vi "S4GUI_001.vi"() -> ()   [LabVIEW 2018] (continued)
            n2258 = call-dynamic "Write ObsType.vi"("error in (no error)"=w5379, "ObsType"=w5365, "Interface in"=w5373) -> ("error out"=w5378:errorcluster, "Interface out"=w5372:refnum<class "Interface.lvclass">)  [unwired: 7 in]
            n2259 = call-dynamic "Write Object.vi"("error in (no error)"=w5378, "Object"=w5364, "Interface in"=w5372) -> ("error out"=w5377:errorcluster, "Interface out"=w5371:refnum<class "Interface.lvclass">)  [unwired: 7 in]
            n2260 = call-dynamic "Write Comments.vi"("error in (no error)"=w5377, "Comments"=w5366, "Interface in"=w5371) -> ("error out"=w5358:errorcluster, "Interface out"=w5357:refnum<class "Interface.lvclass">)  [unwired: 7 in]
            n2261 = call-dynamic "Write Observer.vi"("error in (no error)"=w5358, "Observer"=w5363, "Interface in"=w5357) -> ("error out"=w5359:errorcluster, "Interface out"=w5360:refnum<class "Interface.lvclass">)  [unwired: 7 in]
            n2262 = call-dynamic "Write Interface.vi"("error in (no error)"=w5359, "Interface.lvclass"=w5360, "Channel in"=w5374) -> ("error out"=w5352:errorcluster, "Channel out"=w5353:refnum<class "Channel.lvclass">)  [unwired: 7 in]
            n2263 = call-dynamic "Read State Machine.vi"("error in (no error)"=w5352, "Device in"=w5353) -> ("error out"=w5356:errorcluster, "State Machine.lvclass"=w5349:refnum<class "State Machine.lvclass">, "Device out"=w5351:refnum<class "Channel.lvclass">)  [unwired: 7 in]
            n2264 = call "Next State.vi"("error in (no error)"=w5356, "New_State"=12, "State Machine in"=w5349) -> ("error out"=w5355:errorcluster, "State Machine out"=w5348:refnum<class "State Machine.lvclass">)  [unwired: 7 in]
            n2265 = call-dynamic "Write State Machine.vi"("error in (no error)"=w5355, "State Machine.lvclass"=w5348, "Device in"=w5351) -> ("error out"=w5347:errorcluster, "Device out"=w5350:refnum<class "Channel.lvclass">)  [unwired: 7 in]
            n2266 = call-dynamic "Write Channel.vi"("error in (no error)"=w5347, "Channel.lvclass"=w5350, "Acquisition in"=w5369) -> ("error out"=w5367:errorcluster, "Acquisition out"=w5368:refnum<class "Acquisition.lvclass">)  [unwired: 7 in]
            n2267 = call-dynamic "Write AcquisitionC.vi"("error in (no error)"=w5367, "Acquisition.lvclass"=w5368, "S4ACS_GUI in"=w5370) -> ("error out"=w5381:errorcluster, "S4ACS_GUI out"=w5382:refnum<class "S4GUI.lvclass">)  [unwired: 7 in]
          }
          frame #3 {
            # "object"
            # "suffix"
            # "obsType"
            n2268 = call-dynamic "Read AcquisitionD.vi"("error in (no error)"=w5426, "S4ACS_GUI in"=w5427) -> ("error out"=w5419:errorcluster, "Acquisition.lvclass"=w5418:refnum<class "Acquisition.lvclass">, "S4ACS_GUI out"=w5413:refnum<class "S4GUI.lvclass">)  [unwired: 7 in]
            n2269 = call-dynamic "Read Channel.vi"("error in (no error)"=w5419, "Acquisition in"=w5418) -> ("error out"=w5386:errorcluster, "Channel.lvclass"=w5388:refnum<class "Channel.lvclass">, "Acquisition out"=w5412:refnum<class "Acquisition.lvclass">)  [unwired: 7 in]
            n2270 = local read "Filter4"() -> (w5389:u8)
            n2271 = call-dynamic "Write Filter.vi"("error in (no error)"=w5386, "Filter"=w5389, "Channel in"=w5388) -> ("error out"=w5385:errorcluster, "Channel out"=w5387:refnum<class "Channel.lvclass">)  [unwired: 7 in]
            n2272 = call-dynamic "Read Interface.vi"("error in (no error)"=w5385, "Channel in"=w5387) -> ("error out"=w5404:errorcluster, "Interface.lvclass"=w5405:refnum<class "Interface.lvclass">, "Channel out"=w5417:refnum<class "Channel.lvclass">)  [unwired: 7 in]
            n2273 = call-dynamic "Write Suffix.vi"("error in (no error)"=w5404, "Suffix"=w5423, "Interface in"=w5405) -> ("error out"=w5422:errorcluster, "Interface out"=w5416:refnum<class "Interface.lvclass">)  [unwired: 7 in]
            n2274 = call-dynamic "Write ObsType.vi"("error in (no error)"=w5422, "ObsType"=w5408, "Interface in"=w5416) -> ("error out"=w5421:errorcluster, "Interface out"=w5415:refnum<class "Interface.lvclass">)  [unwired: 7 in]
            n2275 = call-dynamic "Write Object.vi"("error in (no error)"=w5421, "Object"=w5407, "Interface in"=w5415) -> ("error out"=w5420:errorcluster, "Interface out"=w5414:refnum<class "Interface.lvclass">)  [unwired: 7 in]
            n2276 = call-dynamic "Write Comments.vi"("error in (no error)"=w5420, "Comments"=w5409, "Interface in"=w5414) -> ("error out"=w5403:errorcluster, "Interface out"=w5402:refnum<class "Interface.lvclass">)  [unwired: 7 in]
            n2277 = call-dynamic "Write Observer.vi"("error in (no error)"=w5403, "Observer"=w5406, "Interface in"=w5402) -> ("error out"=w5398:errorcluster, "Interface out"=w5397:refnum<class "Interface.lvclass">)  [unwired: 7 in]
            n2278 = call-dynamic "Write Interface.vi"("error in (no error)"=w5398, "Interface.lvclass"=w5397, "Channel in"=w5417) -> ("error out"=w5393:errorcluster, "Channel out"=w5396:refnum<class "Channel.lvclass">)  [unwired: 7 in]
            n2279 = call-dynamic "Read State Machine.vi"("error in (no error)"=w5393, "Device in"=w5396) -> ("error out"=w5401:errorcluster, "State Machine.lvclass"=w5391:refnum<class "State Machine.lvclass">, "Device out"=w5395:refnum<class "Channel.lvclass">)  [unwired: 7 in]
            n2280 = call "Next State.vi"("error in (no error)"=w5401, "New_State"=12, "State Machine in"=w5391) -> ("error out"=w5400:errorcluster, "State Machine out"=w5390:refnum<class "State Machine.lvclass">)  [unwired: 7 in]
            n2281 = call-dynamic "Write State Machine.vi"("error in (no error)"=w5400, "State Machine.lvclass"=w5390, "Device in"=w5395) -> ("error out"=w5392:errorcluster, "Device out"=w5394:refnum<class "Channel.lvclass">)  [unwired: 7 in]
            n2282 = call-dynamic "Write Channel.vi"("error in (no error)"=w5392, "Channel.lvclass"=w5394, "Acquisition in"=w5412) -> ("error out"=w5410:errorcluster, "Acquisition out"=w5411:refnum<class "Acquisition.lvclass">)  [unwired: 7 in]
            n2283 = call-dynamic "Write AcquisitionD.vi"("error in (no error)"=w5410, "Acquisition.lvclass"=w5411, "S4ACS_GUI in"=w5413) -> ("error out"=w5424:errorcluster, "S4ACS_GUI out"=w5425:refnum<class "S4GUI.lvclass">)  [unwired: 7 in]
          }
        }
      }
      event "object suffix", "dflat suffix", "sflat suffix", "dark suffix", "zero suffix", "focus suffix": Value Change {
        # "Remove todos <\\n> e <space> do sufixo:"
        n2284 = event-data() -> ("NewVal"=w5436:string)  [unwired: 1 in, 5 out]
        n2285 = To Lower Case(string=w5436) -> (all lower case string=w5435:string)
        n2286 = call <vilib>:"Trim Whitespace.vi"("string"=w5435) -> ("trimmed string"=w5434:string)  [unwired: 1 in]
        n2287 = Search and Replace String(replace all?=TRUE ("replace all? (F)"), input string=w5434, search string="\n") -> (result string=w5432:string)  [unwired: 5 in, 3 out]
        n2288 = call <vilib>:"Space Constant.vi"() -> ("String"=w5430:string)
        n2289 = Search and Replace String(replace all?=TRUE ("replace all? (F)"), input string=w5432, search string=w5430) -> (result string=w5433:string)  [unwired: 5 in, 3 out]
        n2290 = stacked-sequence {
          seq-local: [w5472 _ _ _] -> [_ w5530 _ _]
          seq-local: [w5471 _ _ _] -> [_ w5529 _ _]
          seq-local: [_ w5528 _ _] -> [_ _ w5573 _]
          seq-local: [_ w5527 _ _] -> [_ _ w5572 _]
          seq-local: [_ _ w5571 _] -> [_ _ _ w5616]
          seq-local: [_ _ w5570 _] -> [_ _ _ w5615]
          tunnel: w5443 -> [w5484 _ _ _]
          tunnel: w5444 -> [w5483 _ _ _]
          tunnel: [_ _ _ w5614] -> w5438
          tunnel: [_ _ _ w5613] -> w5437
          tunnel: w5433 -> [w5470 w5526 w5569 w5612]
          tunnel: w5441 -> [w5469 w5525 w5555 w5598]
          tunnel: w5439 -> [w5468 w5511 w5554 w5597]
          tunnel: w5442 -> [w5467 w5510 w5553 w5596]
          tunnel: w5440 -> [w5466 w5509 w5552 w5595]
          frame #0 {
            # "observer"
            # "comment"
            # "object"
            # "suffix"
            # "obsType"
            n2291 = call-dynamic "Read AcquisitionA.vi"("error in (no error)"=w5484, "S4ACS_GUI in"=w5483) -> ("error out"=w5482:errorcluster, "Acquisition.lvclass"=w5481:refnum<class "Acquisition.lvclass">, "S4ACS_GUI out"=w5476:refnum<class "S4GUI.lvclass">)  [unwired: 7 in]
            n2292 = call-dynamic "Read Channel.vi"("error in (no error)"=w5482, "Acquisition in"=w5481) -> ("error out"=w5446:errorcluster, "Channel.lvclass"=w5449:refnum<class "Channel.lvclass">, "Acquisition out"=w5475:refnum<class "Acquisition.lvclass">)  [unwired: 7 in]
            n2293 = local read "Filter1"() -> (w5447:u8)
            n2294 = call-dynamic "Write Filter.vi"("error in (no error)"=w5446, "Filter"=w5447, "Channel in"=w5449) -> ("error out"=w5445:errorcluster, "Channel out"=w5448:refnum<class "Channel.lvclass">)  [unwired: 7 in]
            n2295 = call-dynamic "Read Interface.vi"("error in (no error)"=w5445, "Channel in"=w5448) -> ("error out"=w5462:errorcluster, "Interface.lvclass"=w5463:refnum<class "Interface.lvclass">, "Channel out"=w5480:refnum<class "Channel.lvclass">)  [unwired: 7 in]
            n2296 = call-dynamic "Write Suffix.vi"("error in (no error)"=w5462, "Suffix"=w5470, "Interface in"=w5463) -> ("error out"=w5487:errorcluster, "Interface out"=w5479:refnum<class "Interface.lvclass">)  [unwired: 7 in]
            n2297 = call-dynamic "Write ObsType.vi"("error in (no error)"=w5487, "ObsType"=w5468, "Interface in"=w5479) -> ("error out"=w5486:errorcluster, "Interface out"=w5478:refnum<class "Interface.lvclass">)  [unwired: 7 in]
            n2298 = call-dynamic "Write Object.vi"("error in (no error)"=w5486, "Object"=w5467, "Interface in"=w5478) -> ("error out"=w5485:errorcluster, "Interface out"=w5477:refnum<class "Interface.lvclass">)  [unwired: 7 in]
            n2299 = call-dynamic "Write Comments.vi"("error in (no error)"=w5485, "Comments"=w5469, "Interface in"=w5477) -> ("error out"=w5465:errorcluster, "Interface out"=w5464:refnum<class "Interface.lvclass">)  [unwired: 7 in]
            n2300 = call-dynamic "Write Observer.vi"("error in (no error)"=w5465, "Observer"=w5466, "Interface in"=w5464) -> ("error out"=w5460:errorcluster, "Interface out"=w5461:refnum<class "Interface.lvclass">)  [unwired: 7 in]
            n2301 = call-dynamic "Write Interface.vi"("error in (no error)"=w5460, "Interface.lvclass"=w5461, "Channel in"=w5480) -> ("error out"=w5456:errorcluster, "Channel out"=w5459:refnum<class "Channel.lvclass">)  [unwired: 7 in]
            n2302 = call-dynamic "Read State Machine.vi"("error in (no error)"=w5456, "Device in"=w5459) -> ("error out"=w5455:errorcluster, "State Machine.lvclass"=w5453:refnum<class "State Machine.lvclass">, "Device out"=w5458:refnum<class "Channel.lvclass">)  [unwired: 7 in]
            n2303 = call "Next State.vi"("error in (no error)"=w5455, "New_State"=12, "State Machine in"=w5453) -> ("error out"=w5454:errorcluster, "State Machine out"=w5452:refnum<class "State Machine.lvclass">)  [unwired: 7 in]
            n2304 = call-dynamic "Write State Machine.vi"("error in (no error)"=w5454, "State Machine.lvclass"=w5452, "Device in"=w5458) -> ("error out"=w5451:errorcluster, "Device out"=w5457:refnum<class "Channel.lvclass">)  [unwired: 7 in]
            n2305 = call-dynamic "Write Channel.vi"("error in (no error)"=w5451, "Channel.lvclass"=w5457, "Acquisition in"=w5475) -> ("error out"=w5473:errorcluster, "Acquisition out"=w5474:refnum<class "Acquisition.lvclass">)  [unwired: 7 in]
            n2306 = call-dynamic "Write AcquisitionA.vi"("error in (no error)"=w5473, "Acquisition.lvclass"=w5474, "S4ACS_GUI in"=w5476) -> ("error out"=w5471:errorcluster, "S4ACS_GUI out"=w5472:refnum<class "S4GUI.lvclass">)  [unwired: 7 in]
          }
          frame #1 {
            # "object"
            # "suffix"
            # "obsType"
            n2307 = call "Read AcquisitionB.vi"("error in (no error)"=w5529, "S4ACS_GUI in"=w5530) -> ("error out"=w5515:errorcluster, "Acquisition.lvclass"=w5516:refnum<class "Acquisition.lvclass">, "S4ACS_GUI out"=w5521:refnum<class "S4GUI.lvclass">)  [unwired: 7 in]
            n2308 = call-dynamic "Read Channel.vi"("error in (no error)"=w5515, "Acquisition in"=w5516) -> ("error out"=w5489:errorcluster, "Channel.lvclass"=w5491:refnum<class "Channel.lvclass">, "Acquisition out"=w5522:refnum<class "Acquisition.lvclass">)  [unwired: 7 in]
            n2309 = local read "Filter2"() -> (w5492:u8)
            n2310 = call-dynamic "Write Filter.vi"("error in (no error)"=w5489, "Filter"=w5492, "Channel in"=w5491) -> ("error out"=w5488:errorcluster, "Channel out"=w5490:refnum<class "Channel.lvclass">)  [unwired: 7 in]
            n2311 = call-dynamic "Read Interface.vi"("error in (no error)"=w5488, "Channel in"=w5490) -> ("error out"=w5503:errorcluster, "Interface.lvclass"=w5504:refnum<class "Interface.lvclass">, "Channel out"=w5517:refnum<class "Channel.lvclass">)  [unwired: 7 in]
            n2312 = call-dynamic "Write Suffix.vi"("error in (no error)"=w5503, "Suffix"=w5526, "Interface in"=w5504) -> ("error out"=w5512:errorcluster, "Interface out"=w5518:refnum<class "Interface.lvclass">)  [unwired: 7 in]
            n2313 = call-dynamic "Write ObsType.vi"("error in (no error)"=w5512, "ObsType"=w5511, "Interface in"=w5518) -> ("error out"=w5513:errorcluster, "Interface out"=w5519:refnum<class "Interface.lvclass">)  [unwired: 7 in]
            n2314 = call-dynamic "Write Object.vi"("error in (no error)"=w5513, "Object"=w5510, "Interface in"=w5519) -> ("error out"=w5514:errorcluster, "Interface out"=w5520:refnum<class "Interface.lvclass">)  [unwired: 7 in]
            n2315 = call-dynamic "Write Comments.vi"("error in (no error)"=w5514, "Comments"=w5525, "Interface in"=w5520) -> ("error out"=w5506:errorcluster, "Interface out"=w5505:refnum<class "Interface.lvclass">)  [unwired: 7 in]
            n2316 = call-dynamic "Write Observer.vi"("error in (no error)"=w5506, "Observer"=w5509, "Interface in"=w5505) -> ("error out"=w5507:errorcluster, "Interface out"=w5508:refnum<class "Interface.lvclass">)  [unwired: 7 in]
            n2317 = call-dynamic "Write Interface.vi"("error in (no error)"=w5507, "Interface.lvclass"=w5508, "Channel in"=w5517) -> ("error out"=w5496:errorcluster, "Channel out"=w5497:refnum<class "Channel.lvclass">)  [unwired: 7 in]
            n2318 = call-dynamic "Read State Machine.vi"("error in (no error)"=w5496, "Device in"=w5497) -> ("error out"=w5502:errorcluster, "State Machine.lvclass"=w5500:refnum<class "State Machine.lvclass">, "Device out"=w5495:refnum<class "Channel.lvclass">)  [unwired: 7 in]
            n2319 = call "Next State.vi"("error in (no error)"=w5502, "New_State"=12, "State Machine in"=w5500) -> ("error out"=w5501:errorcluster, "State Machine out"=w5499:refnum<class "State Machine.lvclass">)  [unwired: 7 in]
            n2320 = call-dynamic "Write State Machine.vi"("error in (no error)"=w5501, "State Machine.lvclass"=w5499, "Device in"=w5495) -> ("error out"=w5493:errorcluster, "Device out"=w5494:refnum<class "Channel.lvclass">)  [unwired: 7 in]
            n2321 = call-dynamic "Write Channel.vi"("error in (no error)"=w5493, "Channel.lvclass"=w5494, "Acquisition in"=w5522) -> ("error out"=w5524:errorcluster, "Acquisition out"=w5523:refnum<class "Acquisition.lvclass">)  [unwired: 7 in]
            n2322 = call "Write AcquisitionB.vi"("error in (no error)"=w5524, "Acquisition.lvclass"=w5523, "S4ACS_GUI in"=w5521) -> ("error out"=w5527:errorcluster, "S4ACS_GUI out"=w5528:refnum<class "S4GUI.lvclass">)  [unwired: 7 in]
          }
          frame #2 {
            # "object"
            # "suffix"
            # "obsType"
            n2323 = call-dynamic "Read AcquisitionC.vi"("error in (no error)"=w5572, "S4ACS_GUI in"=w5573) -> ("error out"=w5565:errorcluster, "Acquisition.lvclass"=w5564:refnum<class "Acquisition.lvclass">, "S4ACS_GUI out"=w5559:refnum<class "S4GUI.lvclass">)  [unwired: 7 in]
            n2324 = call-dynamic "Read Channel.vi"("error in (no error)"=w5565, "Acquisition in"=w5564) -> ("error out"=w5532:errorcluster, "Channel.lvclass"=w5534:refnum<class "Channel.lvclass">, "Acquisition out"=w5558:refnum<class "Acquisition.lvclass">)  [unwired: 7 in]
            n2325 = local read "Filter3"() -> (w5535:u8)
            n2326 = call-dynamic "Write Filter.vi"("error in (no error)"=w5532, "Filter"=w5535, "Channel in"=w5534) -> ("error out"=w5531:errorcluster, "Channel out"=w5533:refnum<class "Channel.lvclass">)  [unwired: 7 in]
            n2327 = call-dynamic "Read Interface.vi"("error in (no error)"=w5531, "Channel in"=w5533) -> ("error out"=w5550:errorcluster, "Interface.lvclass"=w5551:refnum<class "Interface.lvclass">, "Channel out"=w5563:refnum<class "Channel.lvclass">)  [unwired: 7 in]
            n2328 = call-dynamic "Write Suffix.vi"("error in (no error)"=w5550, "Suffix"=w5569, "Interface in"=w5551) -> ("error out"=w5568:errorcluster, "Interface out"=w5562:refnum<class "Interface.lvclass">)  [unwired: 7 in]
            n2329 = call-dynamic "Write ObsType.vi"("error in (no error)"=w5568, "ObsType"=w5554, "Interface in"=w5562) -> ("error out"=w5567:errorcluster, "Interface out"=w5561:refnum<class "Interface.lvclass">)  [unwired: 7 in]
            n2330 = call-dynamic "Write Object.vi"("error in (no error)"=w5567, "Object"=w5553, "Interface in"=w5561) -> ("error out"=w5566:errorcluster, "Interface out"=w5560:refnum<class "Interface.lvclass">)  [unwired: 7 in]
            n2331 = call-dynamic "Write Comments.vi"("error in (no error)"=w5566, "Comments"=w5555, "Interface in"=w5560) -> ("error out"=w5547:errorcluster, "Interface out"=w5546:refnum<class "Interface.lvclass">)  [unwired: 7 in]
            n2332 = call-dynamic "Write Observer.vi"("error in (no error)"=w5547, "Observer"=w5552, "Interface in"=w5546) -> ("error out"=w5548:errorcluster, "Interface out"=w5549:refnum<class "Interface.lvclass">)  [unwired: 7 in]
            n2333 = call-dynamic "Write Interface.vi"("error in (no error)"=w5548, "Interface.lvclass"=w5549, "Channel in"=w5563) -> ("error out"=w5541:errorcluster, "Channel out"=w5542:refnum<class "Channel.lvclass">)  [unwired: 7 in]
            n2334 = call-dynamic "Read State Machine.vi"("error in (no error)"=w5541, "Device in"=w5542) -> ("error out"=w5545:errorcluster, "State Machine.lvclass"=w5538:refnum<class "State Machine.lvclass">, "Device out"=w5540:refnum<class "Channel.lvclass">)  [unwired: 7 in]
            n2335 = call "Next State.vi"("error in (no error)"=w5545, "New_State"=12, "State Machine in"=w5538) -> ("error out"=w5544:errorcluster, "State Machine out"=w5537:refnum<class "State Machine.lvclass">)  [unwired: 7 in]
            n2336 = call-dynamic "Write State Machine.vi"("error in (no error)"=w5544, "State Machine.lvclass"=w5537, "Device in"=w5540) -> ("error out"=w5536:errorcluster, "Device out"=w5539:refnum<class "Channel.lvclass">)  [unwired: 7 in]
            n2337 = call-dynamic "Write Channel.vi"("error in (no error)"=w5536, "Channel.lvclass"=w5539, "Acquisition in"=w5558) -> ("error out"=w5556:errorcluster, "Acquisition out"=w5557:refnum<class "Acquisition.lvclass">)  [unwired: 7 in]
            n2338 = call-dynamic "Write AcquisitionC.vi"("error in (no error)"=w5556, "Acquisition.lvclass"=w5557, "S4ACS_GUI in"=w5559) -> ("error out"=w5570:errorcluster, "S4ACS_GUI out"=w5571:refnum<class "S4GUI.lvclass">)  [unwired: 7 in]
          }
          frame #3 {
            # "object"
            # "suffix"
            # "obsType"
            n2339 = call-dynamic "Read AcquisitionD.vi"("error in (no error)"=w5615, "S4ACS_GUI in"=w5616) -> ("error out"=w5608:errorcluster, "Acquisition.lvclass"=w5607:refnum<class "Acquisition.lvclass">, "S4ACS_GUI out"=w5602:refnum<class "S4GUI.lvclass">)  [unwired: 7 in]
            n2340 = call-dynamic "Read Channel.vi"("error in (no error)"=w5608, "Acquisition in"=w5607) -> ("error out"=w5575:errorcluster, "Channel.lvclass"=w5577:refnum<class "Channel.lvclass">, "Acquisition out"=w5601:refnum<class "Acquisition.lvclass">)  [unwired: 7 in]
            n2341 = local read "Filter4"() -> (w5578:u8)
            n2342 = call-dynamic "Write Filter.vi"("error in (no error)"=w5575, "Filter"=w5578, "Channel in"=w5577) -> ("error out"=w5574:errorcluster, "Channel out"=w5576:refnum<class "Channel.lvclass">)  [unwired: 7 in]
            n2343 = call-dynamic "Read Interface.vi"("error in (no error)"=w5574, "Channel in"=w5576) -> ("error out"=w5593:errorcluster, "Interface.lvclass"=w5594:refnum<class "Interface.lvclass">, "Channel out"=w5606:refnum<class "Channel.lvclass">)  [unwired: 7 in]
            n2344 = call-dynamic "Write Suffix.vi"("error in (no error)"=w5593, "Suffix"=w5612, "Interface in"=w5594) -> ("error out"=w5611:errorcluster, "Interface out"=w5605:refnum<class "Interface.lvclass">)  [unwired: 7 in]
            n2345 = call-dynamic "Write ObsType.vi"("error in (no error)"=w5611, "ObsType"=w5597, "Interface in"=w5605) -> ("error out"=w5610:errorcluster, "Interface out"=w5604:refnum<class "Interface.lvclass">)  [unwired: 7 in]
            n2346 = call-dynamic "Write Object.vi"("error in (no error)"=w5610, "Object"=w5596, "Interface in"=w5604) -> ("error out"=w5609:errorcluster, "Interface out"=w5603:refnum<class "Interface.lvclass">)  [unwired: 7 in]
            n2347 = call-dynamic "Write Comments.vi"("error in (no error)"=w5609, "Comments"=w5598, "Interface in"=w5603) -> ("error out"=w5592:errorcluster, "Interface out"=w5591:refnum<class "Interface.lvclass">)  [unwired: 7 in]
            n2348 = call-dynamic "Write Observer.vi"("error in (no error)"=w5592, "Observer"=w5595, "Interface in"=w5591) -> ("error out"=w5587:errorcluster, "Interface out"=w5586:refnum<class "Interface.lvclass">)  [unwired: 7 in]
            n2349 = call-dynamic "Write Interface.vi"("error in (no error)"=w5587, "Interface.lvclass"=w5586, "Channel in"=w5606) -> ("error out"=w5582:errorcluster, "Channel out"=w5585:refnum<class "Channel.lvclass">)  [unwired: 7 in]
            n2350 = call-dynamic "Read State Machine.vi"("error in (no error)"=w5582, "Device in"=w5585) -> ("error out"=w5590:errorcluster, "State Machine.lvclass"=w5580:refnum<class "State Machine.lvclass">, "Device out"=w5584:refnum<class "Channel.lvclass">)  [unwired: 7 in]
            n2351 = call "Next State.vi"("error in (no error)"=w5590, "New_State"=12, "State Machine in"=w5580) -> ("error out"=w5589:errorcluster, "State Machine out"=w5579:refnum<class "State Machine.lvclass">)  [unwired: 7 in]
            n2352 = call-dynamic "Write State Machine.vi"("error in (no error)"=w5589, "State Machine.lvclass"=w5579, "Device in"=w5584) -> ("error out"=w5581:errorcluster, "Device out"=w5583:refnum<class "Channel.lvclass">)  [unwired: 7 in]
            n2353 = call-dynamic "Write Channel.vi"("error in (no error)"=w5581, "Channel.lvclass"=w5583, "Acquisition in"=w5601) -> ("error out"=w5599:errorcluster, "Acquisition out"=w5600:refnum<class "Acquisition.lvclass">)  [unwired: 7 in]
            n2354 = call-dynamic "Write AcquisitionD.vi"("error in (no error)"=w5599, "Acquisition.lvclass"=w5600, "S4ACS_GUI in"=w5602) -> ("error out"=w5613:errorcluster, "S4ACS_GUI out"=w5614:refnum<class "S4GUI.lvclass">)  [unwired: 7 in]
          }
        }
      }
      event "Observer": Value Change {
        n2355 = event-data() -> ("NewVal"=w5617:string)  [unwired: 1 in, 5 out]
        n2356 = disable-structure shown="Enabled" {
          disable-tunnel: w5620 -> [w5635 w5636]
          disable-tunnel: w5617 -> [w5634 _]
          disable-tunnel: [w5633 w5636] -> w5619
          frame Disabled {
            n2357 = String Length(string=w5634) -> (length=w5632:i32)
            n2358 = Equal To 0?(x=w5632) -> (x = 0?=w5631:bool)
            n2359 = Select(t=u32 16777216, s=w5631, f=u32 16777225) -> (s? t:f=w5629:u32)
            n2360 = property on="Observer" class="Str"(error in=w5635, "Text.BGColor"=w5629) -> (error out=w5633:errorcluster)  [unwired: 1 in, 1 out]
          }
          frame Enabled {
            # "Não se usa mais o texto de fundo\ndo controle \"Observer\""
          }
        }
        n2361 = case shown="False" FALSE {
          tunnel: w5627 -> [w5645 w5819]
          tunnel: w5626 -> [w5644 _]
          tunnel: w5625 -> [w5643 _]
          tunnel: w5624 -> [w5642 _]
          tunnel: w5617 -> [w5641 _]
          tunnel: w5623 -> [w5640 _]
          tunnel: [w5639 w5819] -> w5622
          tunnel: [w5638 w5818] -> w5621
          tunnel: w5619 -> [w5637 w5818]
          frame False {
            n2362 = stacked-sequence {
              seq-local: [w5673 _ _ _] -> [_ w5731 _ _]
              seq-local: [w5672 _ _ _] -> [_ w5730 _ _]
              seq-local: [_ w5729 _ _] -> [_ _ w5774 _]
              seq-local: [_ w5728 _ _] -> [_ _ w5773 _]
              seq-local: [_ _ w5772 _] -> [_ _ _ w5817]
              seq-local: [_ _ w5771 _] -> [_ _ _ w5816]
              tunnel: w5637 -> [w5685 _ _ _]
              tunnel: w5645 -> [w5684 _ _ _]
              tunnel: [_ _ _ w5815] -> w5639
              tunnel: [_ _ _ w5814] -> w5638
              tunnel: w5643 -> [w5671 w5727 w5770 w5813]
              tunnel: w5642 -> [w5670 w5726 w5756 w5799]
              tunnel: w5640 -> [w5669 w5712 w5755 w5798]
              tunnel: w5644 -> [w5668 w5711 w5754 w5797]
              tunnel: w5641 -> [w5667 w5710 w5753 w5796]
              frame #0 {
                # "observer"
                # "comment"
                # "object"
                # "suffix"
                # "obsType"
                n2363 = call-dynamic "Read AcquisitionA.vi"("error in (no error)"=w5685, "S4ACS_GUI in"=w5684) -> ("error out"=w5683:errorcluster, "Acquisition.lvclass"=w5682:refnum<class "Acquisition.lvclass">, "S4ACS_GUI out"=w5677:refnum<class "S4GUI.lvclass">)  [unwired: 7 in]
                n2364 = call-dynamic "Read Channel.vi"("error in (no error)"=w5683, "Acquisition in"=w5682) -> ("error out"=w5647:errorcluster, "Channel.lvclass"=w5650:refnum<class "Channel.lvclass">, "Acquisition out"=w5676:refnum<class "Acquisition.lvclass">)  [unwired: 7 in]
                n2365 = local read "Filter1"() -> (w5648:u8)
                n2366 = call-dynamic "Write Filter.vi"("error in (no error)"=w5647, "Filter"=w5648, "Channel in"=w5650) -> ("error out"=w5646:errorcluster, "Channel out"=w5649:refnum<class "Channel.lvclass">)  [unwired: 7 in]
                n2367 = call-dynamic "Read Interface.vi"("error in (no error)"=w5646, "Channel in"=w5649) -> ("error out"=w5663:errorcluster, "Interface.lvclass"=w5664:refnum<class "Interface.lvclass">, "Channel out"=w5681:refnum<class "Channel.lvclass">)  [unwired: 7 in]
                n2368 = call-dynamic "Write Suffix.vi"("error in (no error)"=w5663, "Suffix"=w5671, "Interface in"=w5664) -> ("error out"=w5688:errorcluster, "Interface out"=w5680:refnum<class "Interface.lvclass">)  [unwired: 7 in]
                n2369 = call-dynamic "Write ObsType.vi"("error in (no error)"=w5688, "ObsType"=w5669, "Interface in"=w5680) -> ("error out"=w5687:errorcluster, "Interface out"=w5679:refnum<class "Interface.lvclass">)  [unwired: 7 in]
                n2370 = call-dynamic "Write Object.vi"("error in (no error)"=w5687, "Object"=w5668, "Interface in"=w5679) -> ("error out"=w5686:errorcluster, "Interface out"=w5678:refnum<class "Interface.lvclass">)  [unwired: 7 in]
                n2371 = call-dynamic "Write Comments.vi"("error in (no error)"=w5686, "Comments"=w5670, "Interface in"=w5678) -> ("error out"=w5666:errorcluster, "Interface out"=w5665:refnum<class "Interface.lvclass">)  [unwired: 7 in]
                n2372 = call-dynamic "Write Observer.vi"("error in (no error)"=w5666, "Observer"=w5667, "Interface in"=w5665) -> ("error out"=w5661:errorcluster, "Interface out"=w5662:refnum<class "Interface.lvclass">)  [unwired: 7 in]
                n2373 = call-dynamic "Write Interface.vi"("error in (no error)"=w5661, "Interface.lvclass"=w5662, "Channel in"=w5681) -> ("error out"=w5657:errorcluster, "Channel out"=w5660:refnum<class "Channel.lvclass">)  [unwired: 7 in]
                n2374 = call-dynamic "Read State Machine.vi"("error in (no error)"=w5657, "Device in"=w5660) -> ("error out"=w5656:errorcluster, "State Machine.lvclass"=w5654:refnum<class "State Machine.lvclass">, "Device out"=w5659:refnum<class "Channel.lvclass">)  [unwired: 7 in]
                n2375 = call "Next State.vi"("error in (no error)"=w5656, "New_State"=12, "State Machine in"=w5654) -> ("error out"=w5655:errorcluster, "State Machine out"=w5653:refnum<class "State Machine.lvclass">)  [unwired: 7 in]
                n2376 = call-dynamic "Write State Machine.vi"("error in (no error)"=w5655, "State Machine.lvclass"=w5653, "Device in"=w5659) -> ("error out"=w5652:errorcluster, "Device out"=w5658:refnum<class "Channel.lvclass">)  [unwired: 7 in]
                n2377 = call-dynamic "Write Channel.vi"("error in (no error)"=w5652, "Channel.lvclass"=w5658, "Acquisition in"=w5676) -> ("error out"=w5674:errorcluster, "Acquisition out"=w5675:refnum<class "Acquisition.lvclass">)  [unwired: 7 in]
                n2378 = call-dynamic "Write AcquisitionA.vi"("error in (no error)"=w5674, "Acquisition.lvclass"=w5675, "S4ACS_GUI in"=w5677) -> ("error out"=w5672:errorcluster, "S4ACS_GUI out"=w5673:refnum<class "S4GUI.lvclass">)  [unwired: 7 in]
              }
              frame #1 {
                # "object"
                # "suffix"
                # "obsType"
                n2379 = call "Read AcquisitionB.vi"("error in (no error)"=w5730, "S4ACS_GUI in"=w5731) -> ("error out"=w5716:errorcluster, "Acquisition.lvclass"=w5717:refnum<class "Acquisition.lvclass">, "S4ACS_GUI out"=w5722:refnum<class "S4GUI.lvclass">)  [unwired: 7 in]
                n2380 = call-dynamic "Read Channel.vi"("error in (no error)"=w5716, "Acquisition in"=w5717) -> ("error out"=w5690:errorcluster, "Channel.lvclass"=w5692:refnum<class "Channel.lvclass">, "Acquisition out"=w5723:refnum<class "Acquisition.lvclass">)  [unwired: 7 in]
                n2381 = local read "Filter2"() -> (w5693:u8)
                n2382 = call-dynamic "Write Filter.vi"("error in (no error)"=w5690, "Filter"=w5693, "Channel in"=w5692) -> ("error out"=w5689:errorcluster, "Channel out"=w5691:refnum<class "Channel.lvclass">)  [unwired: 7 in]
                n2383 = call-dynamic "Read Interface.vi"("error in (no error)"=w5689, "Channel in"=w5691) -> ("error out"=w5704:errorcluster, "Interface.lvclass"=w5705:refnum<class "Interface.lvclass">, "Channel out"=w5718:refnum<class "Channel.lvclass">)  [unwired: 7 in]
                n2384 = call-dynamic "Write Suffix.vi"("error in (no error)"=w5704, "Suffix"=w5727, "Interface in"=w5705) -> ("error out"=w5713:errorcluster, "Interface out"=w5719:refnum<class "Interface.lvclass">)  [unwired: 7 in]
                n2385 = call-dynamic "Write ObsType.vi"("error in (no error)"=w5713, "ObsType"=w5712, "Interface in"=w5719) -> ("error out"=w5714:errorcluster, "Interface out"=w5720:refnum<class "Interface.lvclass">)  [unwired: 7 in]
                n2386 = call-dynamic "Write Object.vi"("error in (no error)"=w5714, "Object"=w5711, "Interface in"=w5720) -> ("error out"=w5715:errorcluster, "Interface out"=w5721:refnum<class "Interface.lvclass">)  [unwired: 7 in]
                n2387 = call-dynamic "Write Comments.vi"("error in (no error)"=w5715, "Comments"=w5726, "Interface in"=w5721) -> ("error out"=w5707:errorcluster, "Interface out"=w5706:refnum<class "Interface.lvclass">)  [unwired: 7 in]
                n2388 = call-dynamic "Write Observer.vi"("error in (no error)"=w5707, "Observer"=w5710, "Interface in"=w5706) -> ("error out"=w5708:errorcluster, "Interface out"=w5709:refnum<class "Interface.lvclass">)  [unwired: 7 in]
                n2389 = call-dynamic "Write Interface.vi"("error in (no error)"=w5708, "Interface.lvclass"=w5709, "Channel in"=w5718) -> ("error out"=w5697:errorcluster, "Channel out"=w5698:refnum<class "Channel.lvclass">)  [unwired: 7 in]
                n2390 = call-dynamic "Read State Machine.vi"("error in (no error)"=w5697, "Device in"=w5698) -> ("error out"=w5703:errorcluster, "State Machine.lvclass"=w5701:refnum<class "State Machine.lvclass">, "Device out"=w5696:refnum<class "Channel.lvclass">)  [unwired: 7 in]
                n2391 = call "Next State.vi"("error in (no error)"=w5703, "New_State"=12, "State Machine in"=w5701) -> ("error out"=w5702:errorcluster, "State Machine out"=w5700:refnum<class "State Machine.lvclass">)  [unwired: 7 in]
                n2392 = call-dynamic "Write State Machine.vi"("error in (no error)"=w5702, "State Machine.lvclass"=w5700, "Device in"=w5696) -> ("error out"=w5694:errorcluster, "Device out"=w5695:refnum<class "Channel.lvclass">)  [unwired: 7 in]
                n2393 = call-dynamic "Write Channel.vi"("error in (no error)"=w5694, "Channel.lvclass"=w5695, "Acquisition in"=w5723) -> ("error out"=w5725:errorcluster, "Acquisition out"=w5724:refnum<class "Acquisition.lvclass">)  [unwired: 7 in]
                n2394 = call "Write AcquisitionB.vi"("error in (no error)"=w5725, "Acquisition.lvclass"=w5724, "S4ACS_GUI in"=w5722) -> ("error out"=w5728:errorcluster, "S4ACS_GUI out"=w5729:refnum<class "S4GUI.lvclass">)  [unwired: 7 in]
              }
              frame #2 {
                # "object"
                # "suffix"
                # "obsType"
                n2395 = call-dynamic "Read AcquisitionC.vi"("error in (no error)"=w5773, "S4ACS_GUI in"=w5774) -> ("error out"=w5766:errorcluster, "Acquisition.lvclass"=w5765:refnum<class "Acquisition.lvclass">, "S4ACS_GUI out"=w5760:refnum<class "S4GUI.lvclass">)  [unwired: 7 in]
                n2396 = call-dynamic "Read Channel.vi"("error in (no error)"=w5766, "Acquisition in"=w5765) -> ("error out"=w5733:errorcluster, "Channel.lvclass"=w5735:refnum<class "Channel.lvclass">, "Acquisition out"=w5759:refnum<class "Acquisition.lvclass">)  [unwired: 7 in]
                n2397 = local read "Filter3"() -> (w5736:u8)
                n2398 = call-dynamic "Write Filter.vi"("error in (no error)"=w5733, "Filter"=w5736, "Channel in"=w5735) -> ("error out"=w5732:errorcluster, "Channel out"=w5734:refnum<class "Channel.lvclass">)  [unwired: 7 in]
                n2399 = call-dynamic "Read Interface.vi"("error in (no error)"=w5732, "Channel in"=w5734) -> ("error out"=w5751:errorcluster, "Interface.lvclass"=w5752:refnum<class "Interface.lvclass">, "Channel out"=w5764:refnum<class "Channel.lvclass">)  [unwired: 7 in]
                n2400 = call-dynamic "Write Suffix.vi"("error in (no error)"=w5751, "Suffix"=w5770, "Interface in"=w5752) -> ("error out"=w5769:errorcluster, "Interface out"=w5763:refnum<class "Interface.lvclass">)  [unwired: 7 in]
                n2401 = call-dynamic "Write ObsType.vi"("error in (no error)"=w5769, "ObsType"=w5755, "Interface in"=w5763) -> ("error out"=w5768:errorcluster, "Interface out"=w5762:refnum<class "Interface.lvclass">)  [unwired: 7 in]
                n2402 = call-dynamic "Write Object.vi"("error in (no error)"=w5768, "Object"=w5754, "Interface in"=w5762) -> ("error out"=w5767:errorcluster, "Interface out"=w5761:refnum<class "Interface.lvclass">)  [unwired: 7 in]
                n2403 = call-dynamic "Write Comments.vi"("error in (no error)"=w5767, "Comments"=w5756, "Interface in"=w5761) -> ("error out"=w5748:errorcluster, "Interface out"=w5747:refnum<class "Interface.lvclass">)  [unwired: 7 in]
                n2404 = call-dynamic "Write Observer.vi"("error in (no error)"=w5748, "Observer"=w5753, "Interface in"=w5747) -> ("error out"=w5749:errorcluster, "Interface out"=w5750:refnum<class "Interface.lvclass">)  [unwired: 7 in]
                n2405 = call-dynamic "Write Interface.vi"("error in (no error)"=w5749, "Interface.lvclass"=w5750, "Channel in"=w5764) -> ("error out"=w5742:errorcluster, "Channel out"=w5743:refnum<class "Channel.lvclass">)  [unwired: 7 in]
                n2406 = call-dynamic "Read State Machine.vi"("error in (no error)"=w5742, "Device in"=w5743) -> ("error out"=w5746:errorcluster, "State Machine.lvclass"=w5739:refnum<class "State Machine.lvclass">, "Device out"=w5741:refnum<class "Channel.lvclass">)  [unwired: 7 in]
                n2407 = call "Next State.vi"("error in (no error)"=w5746, "New_State"=12, "State Machine in"=w5739) -> ("error out"=w5745:errorcluster, "State Machine out"=w5738:refnum<class "State Machine.lvclass">)  [unwired: 7 in]
                n2408 = call-dynamic "Write State Machine.vi"("error in (no error)"=w5745, "State Machine.lvclass"=w5738, "Device in"=w5741) -> ("error out"=w5737:errorcluster, "Device out"=w5740:refnum<class "Channel.lvclass">)  [unwired: 7 in]
                n2409 = call-dynamic "Write Channel.vi"("error in (no error)"=w5737, "Channel.lvclass"=w5740, "Acquisition in"=w5759) -> ("error out"=w5757:errorcluster, "Acquisition out"=w5758:refnum<class "Acquisition.lvclass">)  [unwired: 7 in]
                n2410 = call-dynamic "Write AcquisitionC.vi"("error in (no error)"=w5757, "Acquisition.lvclass"=w5758, "S4ACS_GUI in"=w5760) -> ("error out"=w5771:errorcluster, "S4ACS_GUI out"=w5772:refnum<class "S4GUI.lvclass">)  [unwired: 7 in]
              }
              frame #3 {
                # "object"
                # "suffix"
                # "obsType"
                n2411 = call-dynamic "Read AcquisitionD.vi"("error in (no error)"=w5816, "S4ACS_GUI in"=w5817) -> ("error out"=w5809:errorcluster, "Acquisition.lvclass"=w5808:refnum<class "Acquisition.lvclass">, "S4ACS_GUI out"=w5803:refnum<class "S4GUI.lvclass">)  [unwired: 7 in]
                n2412 = call-dynamic "Read Channel.vi"("error in (no error)"=w5809, "Acquisition in"=w5808) -> ("error out"=w5776:errorcluster, "Channel.lvclass"=w5778:refnum<class "Channel.lvclass">, "Acquisition out"=w5802:refnum<class "Acquisition.lvclass">)  [unwired: 7 in]
                n2413 = local read "Filter4"() -> (w5779:u8)
                n2414 = call-dynamic "Write Filter.vi"("error in (no error)"=w5776, "Filter"=w5779, "Channel in"=w5778) -> ("error out"=w5775:errorcluster, "Channel out"=w5777:refnum<class "Channel.lvclass">)  [unwired: 7 in]
                n2415 = call-dynamic "Read Interface.vi"("error in (no error)"=w5775, "Channel in"=w5777) -> ("error out"=w5794:errorcluster, "Interface.lvclass"=w5795:refnum<class "Interface.lvclass">, "Channel out"=w5807:refnum<class "Channel.lvclass">)  [unwired: 7 in]
                n2416 = call-dynamic "Write Suffix.vi"("error in (no error)"=w5794, "Suffix"=w5813, "Interface in"=w5795) -> ("error out"=w5812:errorcluster, "Interface out"=w5806:refnum<class "Interface.lvclass">)  [unwired: 7 in]
                n2417 = call-dynamic "Write ObsType.vi"("error in (no error)"=w5812, "ObsType"=w5798, "Interface in"=w5806) -> ("error out"=w5811:errorcluster, "Interface out"=w5805:refnum<class "Interface.lvclass">)  [unwired: 7 in]
                n2418 = call-dynamic "Write Object.vi"("error in (no error)"=w5811, "Object"=w5797, "Interface in"=w5805) -> ("error out"=w5810:errorcluster, "Interface out"=w5804:refnum<class "Interface.lvclass">)  [unwired: 7 in]
                n2419 = call-dynamic "Write Comments.vi"("error in (no error)"=w5810, "Comments"=w5799, "Interface in"=w5804) -> ("error out"=w5793:errorcluster, "Interface out"=w5792:refnum<class "Interface.lvclass">)  [unwired: 7 in]
                n2420 = call-dynamic "Write Observer.vi"("error in (no error)"=w5793, "Observer"=w5796, "Interface in"=w5792) -> ("error out"=w5788:errorcluster, "Interface out"=w5787:refnum<class "Interface.lvclass">)  [unwired: 7 in]
                n2421 = call-dynamic "Write Interface.vi"("error in (no error)"=w5788, "Interface.lvclass"=w5787, "Channel in"=w5807) -> ("error out"=w5783:errorcluster, "Channel out"=w5786:refnum<class "Channel.lvclass">)  [unwired: 7 in]
                n2422 = call-dynamic "Read State Machine.vi"("error in (no error)"=w5783, "Device in"=w5786) -> ("error out"=w5791:errorcluster, "State Machine.lvclass"=w5781:refnum<class "State Machine.lvclass">, "Device out"=w5785:refnum<class "Channel.lvclass">)  [unwired: 7 in]
                n2423 = call "Next State.vi"("error in (no error)"=w5791, "New_State"=12, "State Machine in"=w5781) -> ("error out"=w5790:errorcluster, "State Machine out"=w5780:refnum<class "State Machine.lvclass">)  [unwired: 7 in]
                n2424 = call-dynamic "Write State Machine.vi"("error in (no error)"=w5790, "State Machine.lvclass"=w5780, "Device in"=w5785) -> ("error out"=w5782:errorcluster, "Device out"=w5784:refnum<class "Channel.lvclass">)  [unwired: 7 in]
                n2425 = call-dynamic "Write Channel.vi"("error in (no error)"=w5782, "Channel.lvclass"=w5784, "Acquisition in"=w5802) -> ("error out"=w5800:errorcluster, "Acquisition out"=w5801:refnum<class "Acquisition.lvclass">)  [unwired: 7 in]
                n2426 = call-dynamic "Write AcquisitionD.vi"("error in (no error)"=w5800, "Acquisition.lvclass"=w5801, "S4ACS_GUI in"=w5803) -> ("error out"=w5814:errorcluster, "S4ACS_GUI out"=w5815:refnum<class "S4GUI.lvclass">)  [unwired: 7 in]
              }
            }
          }
          frame True {
          }
        }
      }
      event "Observer": Mouse Enter {
        n2427 = event-data() -> ()  [unwired: 1 in, 4 out]
        n2428 = disable-structure shown="Enabled" {
          disable-tunnel: [w5825 w5828] -> w5821
          disable-tunnel: w5820 -> [w5823 w5828]
          frame Disabled {
            n2429 = property on="Observer" class="Str"() -> ("Value"=w5824:string)  [unwired: 2 in, 2 out]
            n2430 = String Length(string=w5824) -> (length=w5827:i32)
            n2431 = Equal To 0?(x=w5827) -> (x = 0?=w5826:bool)
            n2432 = property on="Observer" class="Str"(error in=w5823, "Caption.Visible"=w5826) -> (error out=w5825:errorcluster)  [unwired: 1 in, 1 out]
          }
          frame Enabled {
            # "Não se usa mais o texto de fundo\ndo controle \"Observer\""
          }
        }
      }
      event "Filter1", "Filter2", "Filter3", "Filter4": Value Change {
        n2433 = event-data() -> ()  [unwired: 1 in, 6 out]
        n2434 = stacked-sequence {
          seq-local: [w5865 _ _ _] -> [_ w5923 _ _]
          seq-local: [w5864 _ _ _] -> [_ w5922 _ _]
          seq-local: [_ w5921 _ _] -> [_ _ w5966 _]
          seq-local: [_ w5920 _ _] -> [_ _ w5965 _]
          seq-local: [_ _ w5964 _] -> [_ _ _ w6009]
          seq-local: [_ _ w5963 _] -> [_ _ _ w6008]
          tunnel: w5836 -> [w5877 _ _ _]
          tunnel: w5837 -> [w5876 _ _ _]
          tunnel: [_ _ _ w6007] -> w5830
          tunnel: [_ _ _ w6006] -> w5829
          tunnel: w5834 -> [w5863 w5919 w5962 w6005]
          tunnel: w5833 -> [w5862 w5918 w5948 w5991]
          tunnel: w5831 -> [w5861 w5904 w5947 w5990]
          tunnel: w5835 -> [w5860 w5903 w5946 w5989]
          tunnel: w5832 -> [w5859 w5902 w5945 w5988]
          frame #0 {
            # "observer"
            # "comment"
            # "object"
            # "suffix"
            # "obsType"
            n2435 = call-dynamic "Read AcquisitionA.vi"("error in (no error)"=w5877, "S4ACS_GUI in"=w5876) -> ("error out"=w5875:errorcluster, "Acquisition.lvclass"=w5874:refnum<class "Acquisition.lvclass">, "S4ACS_GUI out"=w5869:refnum<class "S4GUI.lvclass">)  [unwired: 7 in]
            n2436 = call-dynamic "Read Channel.vi"("error in (no error)"=w5875, "Acquisition in"=w5874) -> ("error out"=w5839:errorcluster, "Channel.lvclass"=w5842:refnum<class "Channel.lvclass">, "Acquisition out"=w5868:refnum<class "Acquisition.lvclass">)  [unwired: 7 in]
            n2437 = local read "Filter1"() -> (w5840:u8)
            n2438 = call-dynamic "Write Filter.vi"("error in (no error)"=w5839, "Filter"=w5840, "Channel in"=w5842) -> ("error out"=w5838:errorcluster, "Channel out"=w5841:refnum<class "Channel.lvclass">)  [unwired: 7 in]
            n2439 = call-dynamic "Read Interface.vi"("error in (no error)"=w5838, "Channel in"=w5841) -> ("error out"=w5855:errorcluster, "Interface.lvclass"=w5856:refnum<class "Interface.lvclass">, "Channel out"=w5873:refnum<class "Channel.lvclass">)  [unwired: 7 in]
            n2440 = call-dynamic "Write Suffix.vi"("error in (no error)"=w5855, "Suffix"=w5863, "Interface in"=w5856) -> ("error out"=w5880:errorcluster, "Interface out"=w5872:refnum<class "Interface.lvclass">)  [unwired: 7 in]
            n2441 = call-dynamic "Write ObsType.vi"("error in (no error)"=w5880, "ObsType"=w5861, "Interface in"=w5872) -> ("error out"=w5879:errorcluster, "Interface out"=w5871:refnum<class "Interface.lvclass">)  [unwired: 7 in]
            n2442 = call-dynamic "Write Object.vi"("error in (no error)"=w5879, "Object"=w5860, "Interface in"=w5871) -> ("error out"=w5878:errorcluster, "Interface out"=w5870:refnum<class "Interface.lvclass">)  [unwired: 7 in]
            n2443 = call-dynamic "Write Comments.vi"("error in (no error)"=w5878, "Comments"=w5862, "Interface in"=w5870) -> ("error out"=w5858:errorcluster, "Interface out"=w5857:refnum<class "Interface.lvclass">)  [unwired: 7 in]
            n2444 = call-dynamic "Write Observer.vi"("error in (no error)"=w5858, "Observer"=w5859, "Interface in"=w5857) -> ("error out"=w5853:errorcluster, "Interface out"=w5854:refnum<class "Interface.lvclass">)  [unwired: 7 in]
            n2445 = call-dynamic "Write Interface.vi"("error in (no error)"=w5853, "Interface.lvclass"=w5854, "Channel in"=w5873) -> ("error out"=w5849:errorcluster, "Channel out"=w5852:refnum<class "Channel.lvclass">)  [unwired: 7 in]
            n2446 = call-dynamic "Read State Machine.vi"("error in (no error)"=w5849, "Device in"=w5852) -> ("error out"=w5848:errorcluster, "State Machine.lvclass"=w5846:refnum<class "State Machine.lvclass">, "Device out"=w5851:refnum<class "Channel.lvclass">)  [unwired: 7 in]
            n2447 = call "Next State.vi"("error in (no error)"=w5848, "New_State"=12, "State Machine in"=w5846) -> ("error out"=w5847:errorcluster, "State Machine out"=w5845:refnum<class "State Machine.lvclass">)  [unwired: 7 in]
            n2448 = call-dynamic "Write State Machine.vi"("error in (no error)"=w5847, "State Machine.lvclass"=w5845, "Device in"=w5851) -> ("error out"=w5844:errorcluster, "Device out"=w5850:refnum<class "Channel.lvclass">)  [unwired: 7 in]
            n2449 = call-dynamic "Write Channel.vi"("error in (no error)"=w5844, "Channel.lvclass"=w5850, "Acquisition in"=w5868) -> ("error out"=w5866:errorcluster, "Acquisition out"=w5867:refnum<class "Acquisition.lvclass">)  [unwired: 7 in]
            n2450 = call-dynamic "Write AcquisitionA.vi"("error in (no error)"=w5866, "Acquisition.lvclass"=w5867, "S4ACS_GUI in"=w5869) -> ("error out"=w5864:errorcluster, "S4ACS_GUI out"=w5865:refnum<class "S4GUI.lvclass">)  [unwired: 7 in]
          }
          frame #1 {
            # "object"
            # "suffix"
            # "obsType"
            n2451 = call "Read AcquisitionB.vi"("error in (no error)"=w5922, "S4ACS_GUI in"=w5923) -> ("error out"=w5908:errorcluster, "Acquisition.lvclass"=w5909:refnum<class "Acquisition.lvclass">, "S4ACS_GUI out"=w5914:refnum<class "S4GUI.lvclass">)  [unwired: 7 in]
            n2452 = call-dynamic "Read Channel.vi"("error in (no error)"=w5908, "Acquisition in"=w5909) -> ("error out"=w5882:errorcluster, "Channel.lvclass"=w5884:refnum<class "Channel.lvclass">, "Acquisition out"=w5915:refnum<class "Acquisition.lvclass">)  [unwired: 7 in]
            n2453 = local read "Filter2"() -> (w5885:u8)
            n2454 = call-dynamic "Write Filter.vi"("error in (no error)"=w5882, "Filter"=w5885, "Channel in"=w5884) -> ("error out"=w5881:errorcluster, "Channel out"=w5883:refnum<class "Channel.lvclass">)  [unwired: 7 in]
            n2455 = call-dynamic "Read Interface.vi"("error in (no error)"=w5881, "Channel in"=w5883) -> ("error out"=w5896:errorcluster, "Interface.lvclass"=w5897:refnum<class "Interface.lvclass">, "Channel out"=w5910:refnum<class "Channel.lvclass">)  [unwired: 7 in]
            n2456 = call-dynamic "Write Suffix.vi"("error in (no error)"=w5896, "Suffix"=w5919, "Interface in"=w5897) -> ("error out"=w5905:errorcluster, "Interface out"=w5911:refnum<class "Interface.lvclass">)  [unwired: 7 in]
            n2457 = call-dynamic "Write ObsType.vi"("error in (no error)"=w5905, "ObsType"=w5904, "Interface in"=w5911) -> ("error out"=w5906:errorcluster, "Interface out"=w5912:refnum<class "Interface.lvclass">)  [unwired: 7 in]
            n2458 = call-dynamic "Write Object.vi"("error in (no error)"=w5906, "Object"=w5903, "Interface in"=w5912) -> ("error out"=w5907:errorcluster, "Interface out"=w5913:refnum<class "Interface.lvclass">)  [unwired: 7 in]
            n2459 = call-dynamic "Write Comments.vi"("error in (no error)"=w5907, "Comments"=w5918, "Interface in"=w5913) -> ("error out"=w5899:errorcluster, "Interface out"=w5898:refnum<class "Interface.lvclass">)  [unwired: 7 in]
            n2460 = call-dynamic "Write Observer.vi"("error in (no error)"=w5899, "Observer"=w5902, "Interface in"=w5898) -> ("error out"=w5900:errorcluster, "Interface out"=w5901:refnum<class "Interface.lvclass">)  [unwired: 7 in]
            n2461 = call-dynamic "Write Interface.vi"("error in (no error)"=w5900, "Interface.lvclass"=w5901, "Channel in"=w5910) -> ("error out"=w5889:errorcluster, "Channel out"=w5890:refnum<class "Channel.lvclass">)  [unwired: 7 in]
            n2462 = call-dynamic "Read State Machine.vi"("error in (no error)"=w5889, "Device in"=w5890) -> ("error out"=w5895:errorcluster, "State Machine.lvclass"=w5893:refnum<class "State Machine.lvclass">, "Device out"=w5888:refnum<class "Channel.lvclass">)  [unwired: 7 in]
            n2463 = call "Next State.vi"("error in (no error)"=w5895, "New_State"=12, "State Machine in"=w5893) -> ("error out"=w5894:errorcluster, "State Machine out"=w5892:refnum<class "State Machine.lvclass">)  [unwired: 7 in]
            n2464 = call-dynamic "Write State Machine.vi"("error in (no error)"=w5894, "State Machine.lvclass"=w5892, "Device in"=w5888) -> ("error out"=w5886:errorcluster, "Device out"=w5887:refnum<class "Channel.lvclass">)  [unwired: 7 in]
            n2465 = call-dynamic "Write Channel.vi"("error in (no error)"=w5886, "Channel.lvclass"=w5887, "Acquisition in"=w5915) -> ("error out"=w5917:errorcluster, "Acquisition out"=w5916:refnum<class "Acquisition.lvclass">)  [unwired: 7 in]
            n2466 = call "Write AcquisitionB.vi"("error in (no error)"=w5917, "Acquisition.lvclass"=w5916, "S4ACS_GUI in"=w5914) -> ("error out"=w5920:errorcluster, "S4ACS_GUI out"=w5921:refnum<class "S4GUI.lvclass">)  [unwired: 7 in]
          }
          frame #2 {
            # "object"
            # "suffix"
            # "obsType"
            n2467 = call-dynamic "Read AcquisitionC.vi"("error in (no error)"=w5965, "S4ACS_GUI in"=w5966) -> ("error out"=w5958:errorcluster, "Acquisition.lvclass"=w5957:refnum<class "Acquisition.lvclass">, "S4ACS_GUI out"=w5952:refnum<class "S4GUI.lvclass">)  [unwired: 7 in]
            n2468 = call-dynamic "Read Channel.vi"("error in (no error)"=w5958, "Acquisition in"=w5957) -> ("error out"=w5925:errorcluster, "Channel.lvclass"=w5927:refnum<class "Channel.lvclass">, "Acquisition out"=w5951:refnum<class "Acquisition.lvclass">)  [unwired: 7 in]
            n2469 = local read "Filter3"() -> (w5928:u8)
            n2470 = call-dynamic "Write Filter.vi"("error in (no error)"=w5925, "Filter"=w5928, "Channel in"=w5927) -> ("error out"=w5924:errorcluster, "Channel out"=w5926:refnum<class "Channel.lvclass">)  [unwired: 7 in]
            n2471 = call-dynamic "Read Interface.vi"("error in (no error)"=w5924, "Channel in"=w5926) -> ("error out"=w5943:errorcluster, "Interface.lvclass"=w5944:refnum<class "Interface.lvclass">, "Channel out"=w5956:refnum<class "Channel.lvclass">)  [unwired: 7 in]
            n2472 = call-dynamic "Write Suffix.vi"("error in (no error)"=w5943, "Suffix"=w5962, "Interface in"=w5944) -> ("error out"=w5961:errorcluster, "Interface out"=w5955:refnum<class "Interface.lvclass">)  [unwired: 7 in]
            n2473 = call-dynamic "Write ObsType.vi"("error in (no error)"=w5961, "ObsType"=w5947, "Interface in"=w5955) -> ("error out"=w5960:errorcluster, "Interface out"=w5954:refnum<class "Interface.lvclass">)  [unwired: 7 in]
            n2474 = call-dynamic "Write Object.vi"("error in (no error)"=w5960, "Object"=w5946, "Interface in"=w5954) -> ("error out"=w5959:errorcluster, "Interface out"=w5953:refnum<class "Interface.lvclass">)  [unwired: 7 in]
            n2475 = call-dynamic "Write Comments.vi"("error in (no error)"=w5959, "Comments"=w5948, "Interface in"=w5953) -> ("error out"=w5940:errorcluster, "Interface out"=w5939:refnum<class "Interface.lvclass">)  [unwired: 7 in]
            n2476 = call-dynamic "Write Observer.vi"("error in (no error)"=w5940, "Observer"=w5945, "Interface in"=w5939) -> ("error out"=w5941:errorcluster, "Interface out"=w5942:refnum<class "Interface.lvclass">)  [unwired: 7 in]
            n2477 = call-dynamic "Write Interface.vi"("error in (no error)"=w5941, "Interface.lvclass"=w5942, "Channel in"=w5956) -> ("error out"=w5934:errorcluster, "Channel out"=w5935:refnum<class "Channel.lvclass">)  [unwired: 7 in]
